vi "thcd_chan_stat.vi"(8 "err_in":errorcluster, 9 "thcd_b2r":u32, 10 "thcd_delay":u32=300, 11 "thcd_visa":refnum<visa-resource-name>) -> (0 "thcd_res_4":T2, 1 "thcd_res_3":T2, 2 "thcd_res_2":T2, 3 "thcd_res_1":T2, 4 "thcd_res_str":string, 5 "thcd_st":bool, 6 "err_out":errorcluster, 7 "thcd_visa":refnum<visa-resource-name>)   [LabVIEW 2018]
uses:
  thcd_controls/ctrl_chn_thcd.ctl
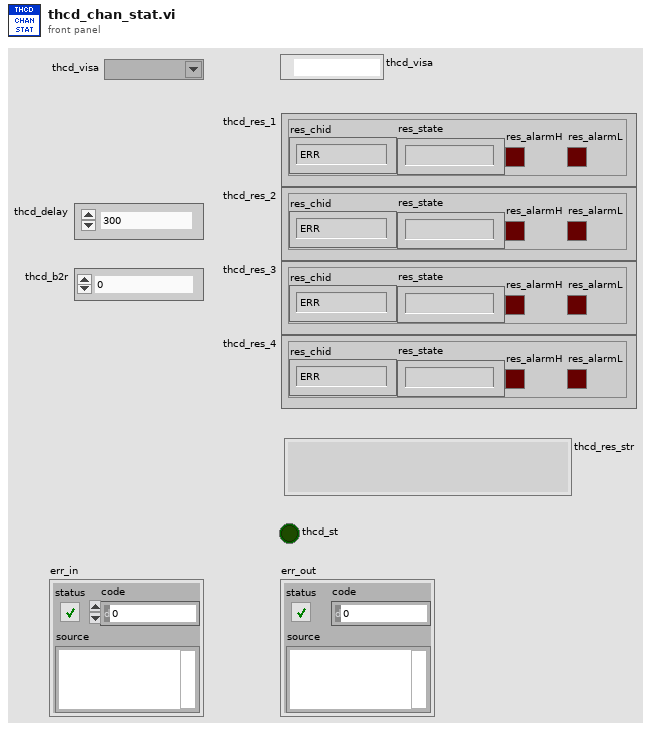
[diagram p1: front panel]
types:
  T1 = typedef "ctrl_chn_thcd.ctl" = enum8{"ERR", "1", "2", "3", "4"}
  T2 = cluster{"res_chid":T1, "res_state":string, "res_alarmH":bool, "res_alarmL":bool}
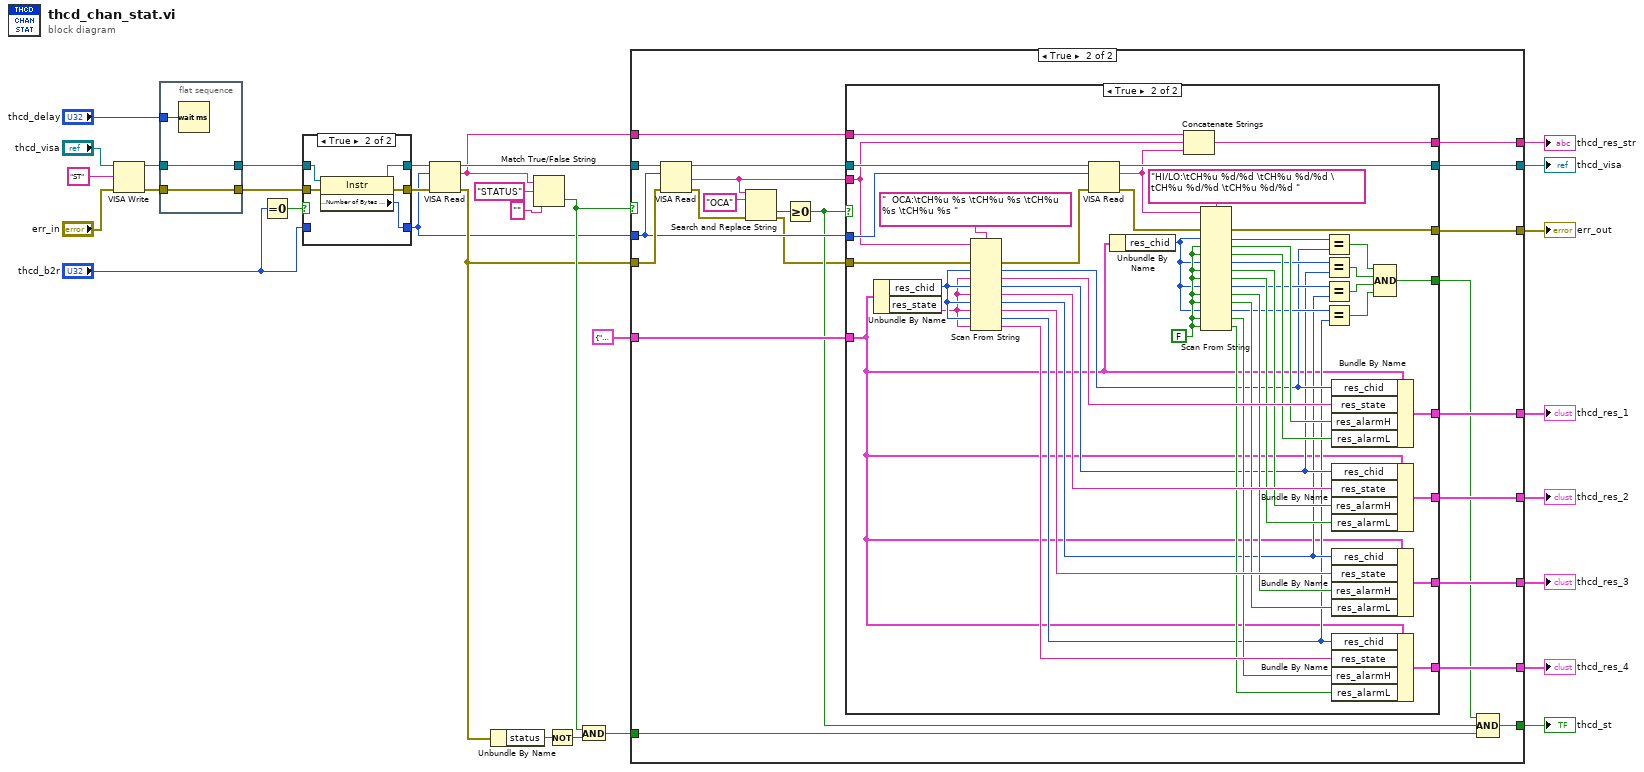
[diagram p0: block diagram]
diagram:
  n1 = VISA Write(VISA resource name="thcd_visa", write buffer="ST" ("format string"), error in (no error)="err_in") -> (VISA resource name out=w30:refnum<visa-resource-name>, error out=w31:errorcluster)  [unwired: 1 out]
  n2 = flat-sequence {
    tunnel: w31 -> [w33]
    tunnel: [w33] -> w24
    tunnel: w30 -> [w32]
    tunnel: [w32] -> w25
    tunnel: "thcd_delay" -> [w34]
    frame #0 {
      n3 = Wait (ms)(milliseconds to wait=w34) -> ()  [unwired: 1 out]
    }
  }
  n4 = Equal To 0?(x="thcd_b2r") -> (x = 0?=w26:bool)
  n5 = case shown="True" w26 {
    tunnel: [w36 w42] -> w23
    tunnel: [w35 w41] -> w22
    tunnel: [w37 w40] -> w10
    tunnel: "thcd_b2r" -> [w37 _]
    tunnel: w25 -> [w36 w39]
    tunnel: w24 -> [w35 w38]
    frame False {
    }
    frame True {
      n6 = property class="Instr"(reference=w39, error in=w38) -> (reference out=w42:refnum<visa-resource-name>, error out=w41:errorcluster, "Serial Settings:Number of Bytes at Serial Port"=w40:u32)
    }
  }
  n7 = VISA Read(VISA resource name=w23, byte count=w10, error in (no error)=w22) -> (VISA resource name out=w11:refnum<visa-resource-name>, read buffer=w1:string, error out=w13:errorcluster)  [unwired: 1 out]
  n8 = Unbundle By Name(w13) -> ("status"=w16:bool)
  n9 = Match True/False String(2:"" ("false string"), 3:"STATUS" ("true string"), 4:w1) -> (0:w14:bool)  [unwired: 1 out]
  n10 = Not(x=w16) -> (.not. x?=w15:bool)
  n11 = And(x=w14, y=w15) -> (x .and. y?=w9:bool)
  n12 = case shown="True" w14 {
    tunnel: [w47 w69] -> w5
    tunnel: T2 {"res_chid"=enum."ERR", "res_state"="", "res_alarmH"=FALSE, "res_alarmL"=FALSE} ("res_1 2") -> [w47 w65]
    tunnel: [w47 w68] -> w6
    tunnel: [w47 w67] -> w4
    tunnel: [w47 w66] -> w3
    tunnel: w13 -> [w46 w62]
    tunnel: [w46 w64] -> w19
    tunnel: w11 -> [w44 w63]
    tunnel: w10 -> [_ w60]
    tunnel: w9 -> [w43 w59]
    tunnel: [w44 w58] -> w8
    tunnel: w1 -> [w45 w57]
    tunnel: [w45 w56] -> w7
    tunnel: [w43 w55] -> w2
    frame False {
    }
    frame True {
      n13 = VISA Read(VISA resource name=w63, byte count=w60, error in (no error)=w62) -> (VISA resource name out=w61:refnum<visa-resource-name>, read buffer=w49:string, error out=w51:errorcluster)  [unwired: 1 out]
      n14 = Search and Replace String(input string=w49, search string="OCA" ("true string"), error in=w51) -> (offset past replacement=w53:i32, error out=w50:errorcluster)  [unwired: 5 in, 2 out]
      n15 = Greater Or Equal To 0?(x=w53) -> (x >= 0?=w52:bool)
      n16 = case shown="True" w52 {
        selector: w52 -> [w70 _]
        tunnel: [w73 w112] -> w69
        tunnel: [w73 w111] -> w68
        tunnel: [w73 w110] -> w67
        tunnel: [w73 w109] -> w66
        tunnel: w65 -> [w73 w80]
        tunnel: [w74 w108] -> w64
        tunnel: w49 -> [_ w100]
        tunnel: w61 -> [w71 w107]
        tunnel: w50 -> [w74 w106]
        tunnel: w60 -> [_ w105]
        tunnel: [w71 w102] -> w58
        tunnel: w57 -> [w72 w101]
        tunnel: [w72 w98] -> w56
        tunnel: [w70 w75] -> w48
        frame False {
        }
        frame True {
          w95 = FALSE
          n17 = Unbundle By Name(w80) -> ("res_chid"=w121:T1, "res_state"=w120:string)
          n18 = Scan From String(format string="  OCA:\tCH%u %s \tCH%u %s \tCH%u %s \tCH%u %s " ("format string 3"), input string=w100, error in=w106, default 1=w121, default 2=w120, default 3=w121, default 4=w120, default 5=w121, default 6=w120, default 7=w121, default 8=w120) -> (error out=w104:errorcluster, output 1=w86:T1, output 2=w118:string, output 3=w85:T1, output 4=w117:string, output 5=w84:T1, output 6=w116:string, output 7=w83:T1, output 8=w115:string)  [unwired: 1 in, 2 out]
          n19 = VISA Read(VISA resource name=w107, byte count=w105, error in (no error)=w104) -> (VISA resource name out=w102:refnum<visa-resource-name>, read buffer=w99:string, error out=w103:errorcluster)  [unwired: 1 out]
          n20 = Unbundle By Name(w80) -> ("res_chid"=w81:T1)
          n21 = Concatenate Strings(w101, w100, w99) -> (w98:string)
          n22 = Scan From String(format string="HI/LO:\tCH%u %d/%d \tCH%u %d/%d \tCH%u %d/%d \tCH%u %d/%d " ("format string 3"), input string=w99, error in=w103, default 1=w81, default 2=w95, default 3=w95, default 4=w81, default 5=w95, default 6=w95, default 7=w81, default 8=w95, default 9=w95, default 10=w81, default 11=w95, default 12=w95) -> (error out=w108:errorcluster, output 1=w90:T1, output 2=w97:bool, output 3=w96:bool, output 4=w89:T1, output 5=w94:bool, output 6=w93:bool, output 7=w88:T1, output 8=w92:bool, output 9=w91:bool, output 10=w87:T1, output 11=w114:bool, output 12=w113:bool)  [unwired: 1 in, 2 out]
          n23 = Equal?(x=w90, y=w86) -> (x = y?=w79:bool)
          n24 = Equal?(x=w89, y=w85) -> (x = y?=w78:bool)
          n25 = Equal?(x=w88, y=w84) -> (x = y?=w77:bool)
          n26 = Equal?(x=w87, y=w83) -> (x = y?=w76:bool)
          n27 = Bundle By Name(cluster=w80, "res_chid"=w86, "res_state"=w118, "res_alarmH"=w97, "res_alarmL"=w96) -> (w112:T2)
          n28 = Bundle By Name(cluster=w80, "res_chid"=w85, "res_state"=w117, "res_alarmH"=w94, "res_alarmL"=w93) -> (w111:T2)
          n29 = Bundle By Name(cluster=w80, "res_chid"=w84, "res_state"=w116, "res_alarmH"=w92, "res_alarmL"=w91) -> (w110:T2)
          n30 = Bundle By Name(cluster=w80, "res_chid"=w83, "res_state"=w115, "res_alarmH"=w114, "res_alarmL"=w113) -> (w109:T2)
          n31 = Compound Arithmetic op=AND(w79, w78, w77, w76) -> (w75:bool)
        }
      }
      n32 = Compound Arithmetic op=AND(w48, w52, w59) -> (w55:bool)
    }
  }
  "err_out" <- w19
  "thcd_visa" <- w8
  "thcd_res_str" <- w7
  "thcd_st" <- w2
  "thcd_res_1" <- w5
  "thcd_res_2" <- w6
  "thcd_res_3" <- w4
  "thcd_res_4" <- w3
